vi "Network Streams Performance Test.vi"() -> ()   [LabVIEW 2021]
uses:
  <vilib>/dex/Stream Element Allocation Mode.ctl
panel:
  out "x-y":dbl format="%#_6p"
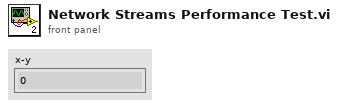
[diagram p1: front panel]
types:
  T1 = typedef "Stream Element Allocation Mode.ctl" = u32
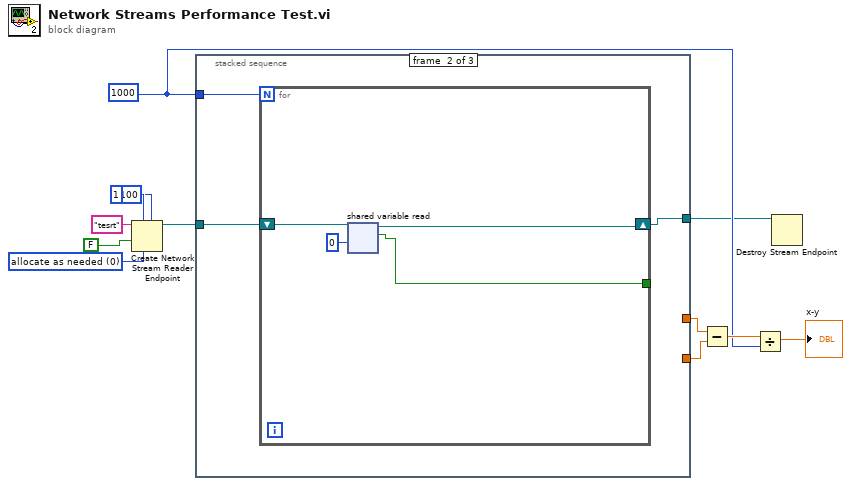
[diagram p0: block diagram]
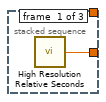
[diagram p2: hidden frame]
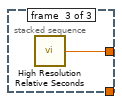
[diagram p3: hidden frame]
diagram:
  w4 = T1 0 items=["allocate as needed", "pre-allocate"] ("element allocation mode")
  w8 = 1000
  n1 = Create Network Stream Reader Endpoint(5:100 ("timeout in ms (-1)"), 6:w4, 7:1 ("reader buffer size"), 9:FALSE, 11:"tesrt" ("reader name")) -> (3:w7:refnum<k21>)  [unwired: 2 in, 1 out]
  n2 = stacked-sequence {
    tunnel: [w13 _ _] -> w12
    tunnel: [_ _ w21] -> w11
    tunnel: w8 -> [_ w16 _]
    tunnel: w7 -> [_ w15 _]
    tunnel: [_ w14 _] -> w2
    frame #0 {
      n3 = call <vilib>:"High Resolution Relative Seconds.vi"() -> ("relative seconds"=w13:dbl)
    }
    frame #1 {
      n4 = for {
        N: w16 -> [_]
        tunnel: [w18] -> _
        shift-right: [w19] -> w14
        shift-left: w15 -> [w20]
        n5 = shared-variable-read(w20, 0 ("timeout ms (-1)")) -> (w19:refnum<k21>, w18:bool)  [unwired: 1 in, 2 out]
      }
    }
    frame #2 {
      n6 = call <vilib>:"High Resolution Relative Seconds.vi"() -> ("relative seconds"=w21:dbl)
    }
  }
  n7 = Subtract(x=w11, y=w12) -> (x-y=w10:dbl)
  n8 = Divide(x=w10, y=w8) -> (x/y=→"x-y":dbl)
  n9 = Destroy Stream Endpoint(11:w2) -> ()  [unwired: 1 in, 1 out]
